vi "op_x2 Functional Test.vi"(0 "ENA1":bool caption="Connection 1 enable", 1 "IP address 1":string="172.16.14.23", 2 "ENA2":bool caption="Connection 2 enable", 3 "IP address 2":string="172.16.14.22", 4 "Operation text Refnum":refnum<vi>, 5 "error tick Refnum":refnum<vi>) -> ()   [LabVIEW 2015, in "VIPM2.lvlib"]
uses:
  VIPM2.lvlib
panel:
  out "Reports 2":string[](array[string])
  out "Reports 1":string[](array[string])
  in  "Close Button":bool
  in  "Execute Button":bool
  in  "Layers 2 cluster":T1(array[cluster]) {"LayerID" format="%x"}
  in  "All Layers 2":bool
  in  "Layers 1 cluster":T1(array[cluster]) {"LayerID" format="%x"}
  in  "All Layers 1":bool
  # "Select the Layers to execute the Functional Test"
  # "Bad pixels masked by software:\n      Chip D9EB: px 14\n      Chip 6B7B: px 60\n      Chip 3A65: px 00, 10, 20, 30, 40"
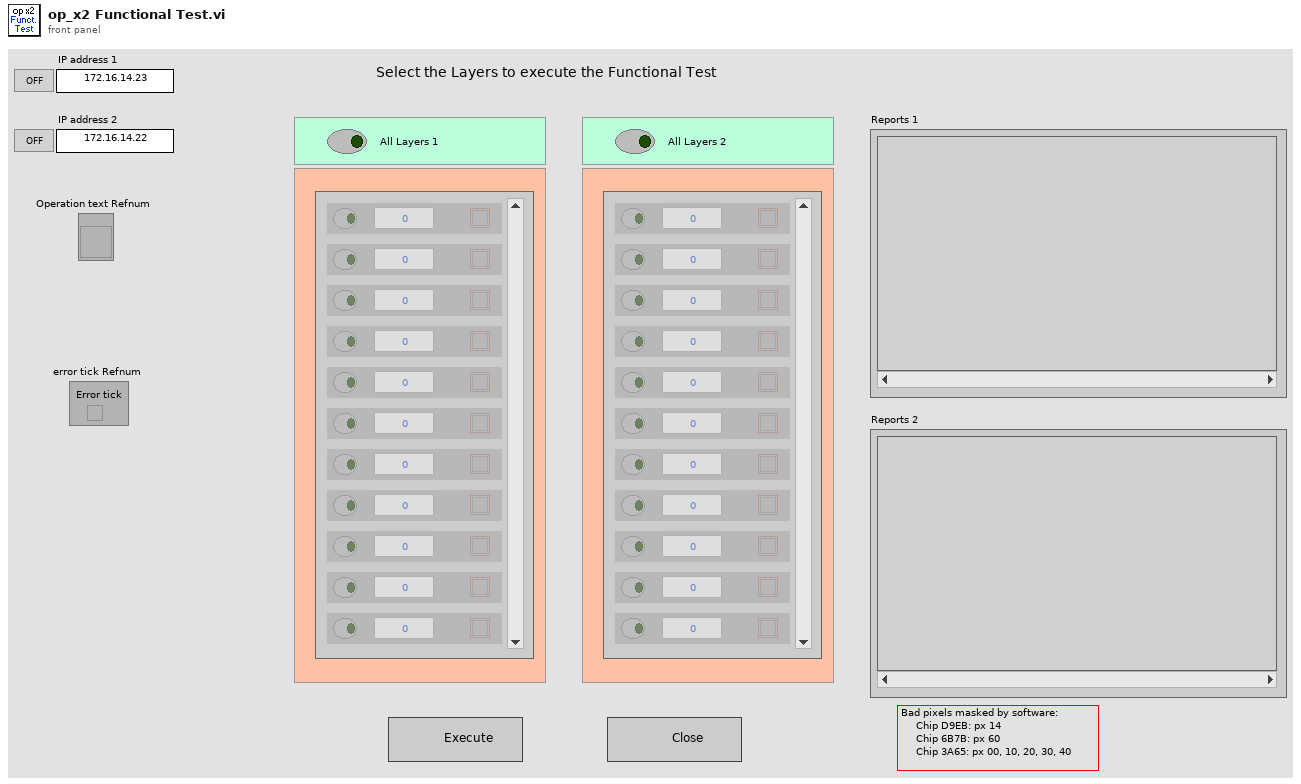
[diagram p1: front panel]
types:
  T1 = cluster{"Button":bool, "LayerID":u32, "Result":bool}[]
  T2 = cluster{"Button":bool, "LayerID":u32, "Result":bool}
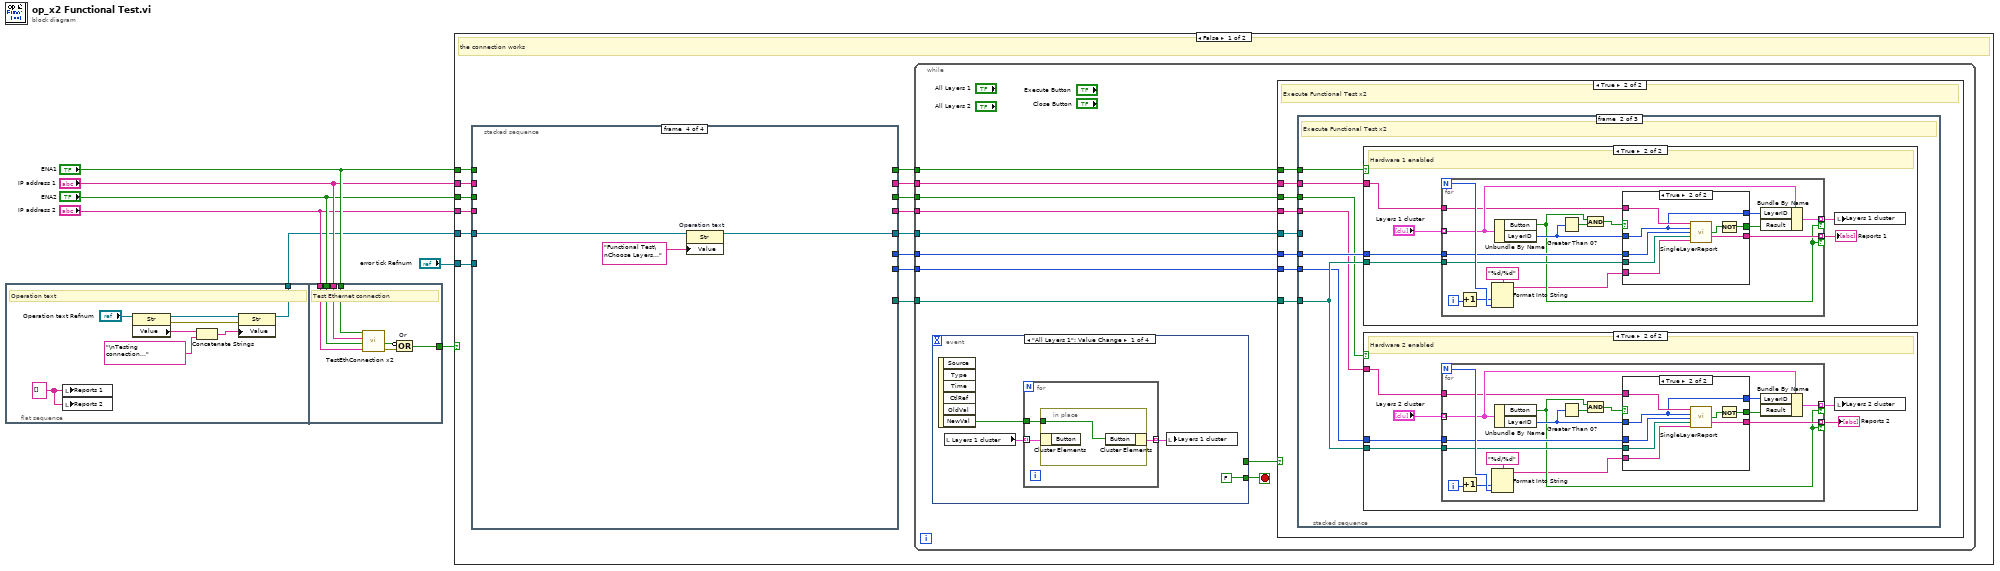
[diagram p0: block diagram]
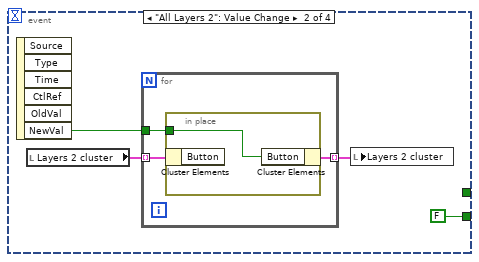
[diagram p2: hidden frame]
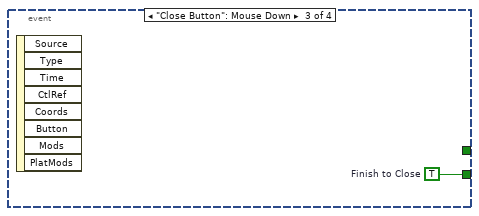
[diagram p3: hidden frame]
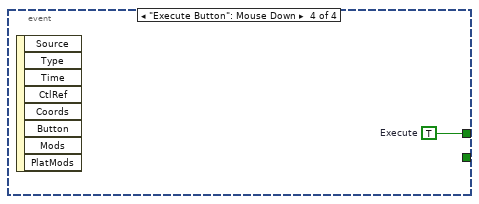
[diagram p4: hidden frame]
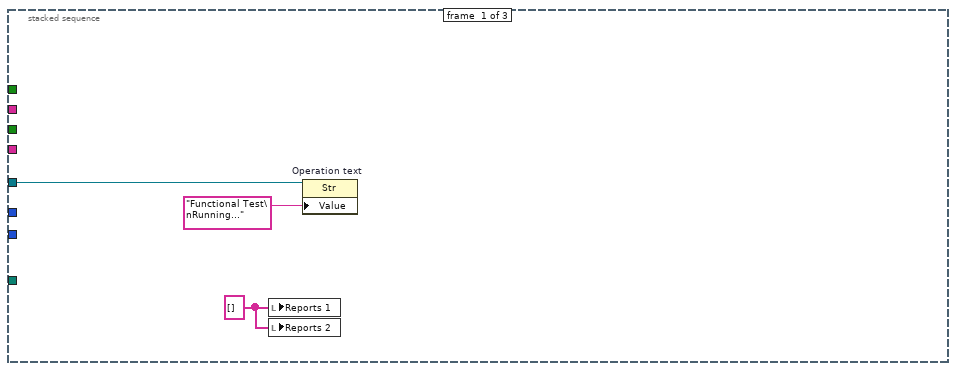
[diagram p6: hidden frame]
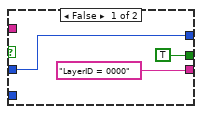
[diagram p8: hidden frame]
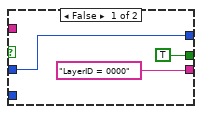
[diagram p10: hidden frame]
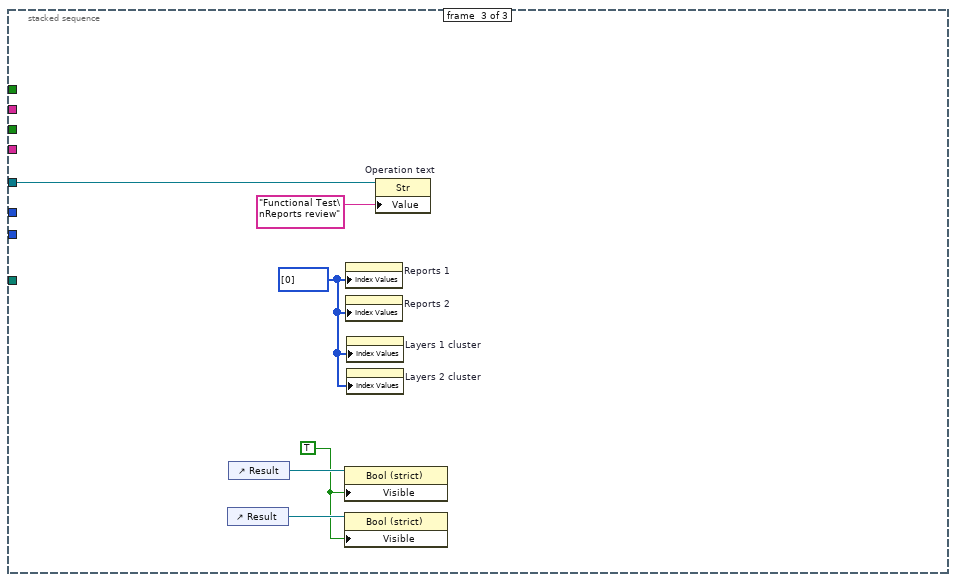
[diagram p11: hidden frame]
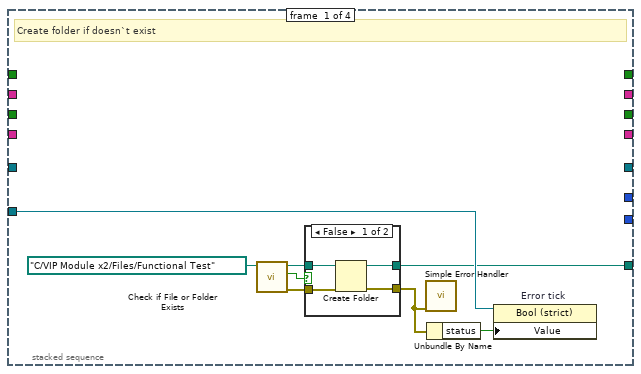
[diagram p12: hidden frame]
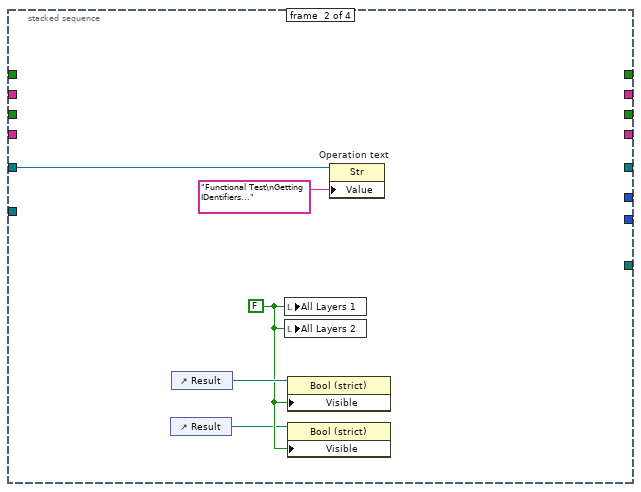
[diagram p14: hidden frame]
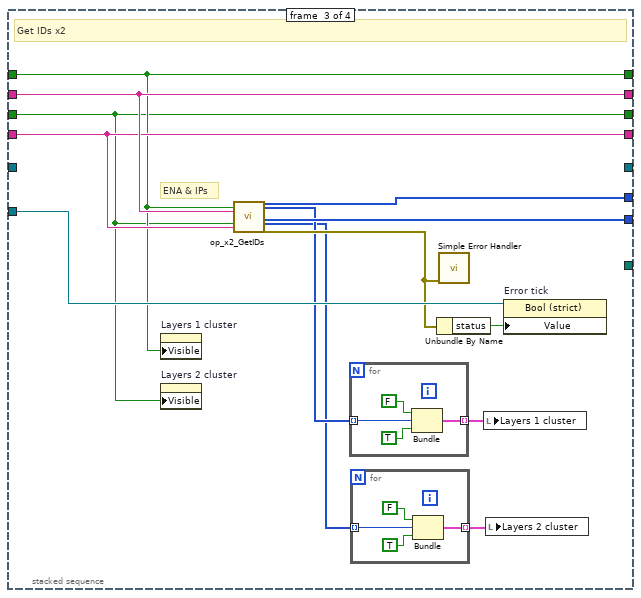
[diagram p15: hidden frame]
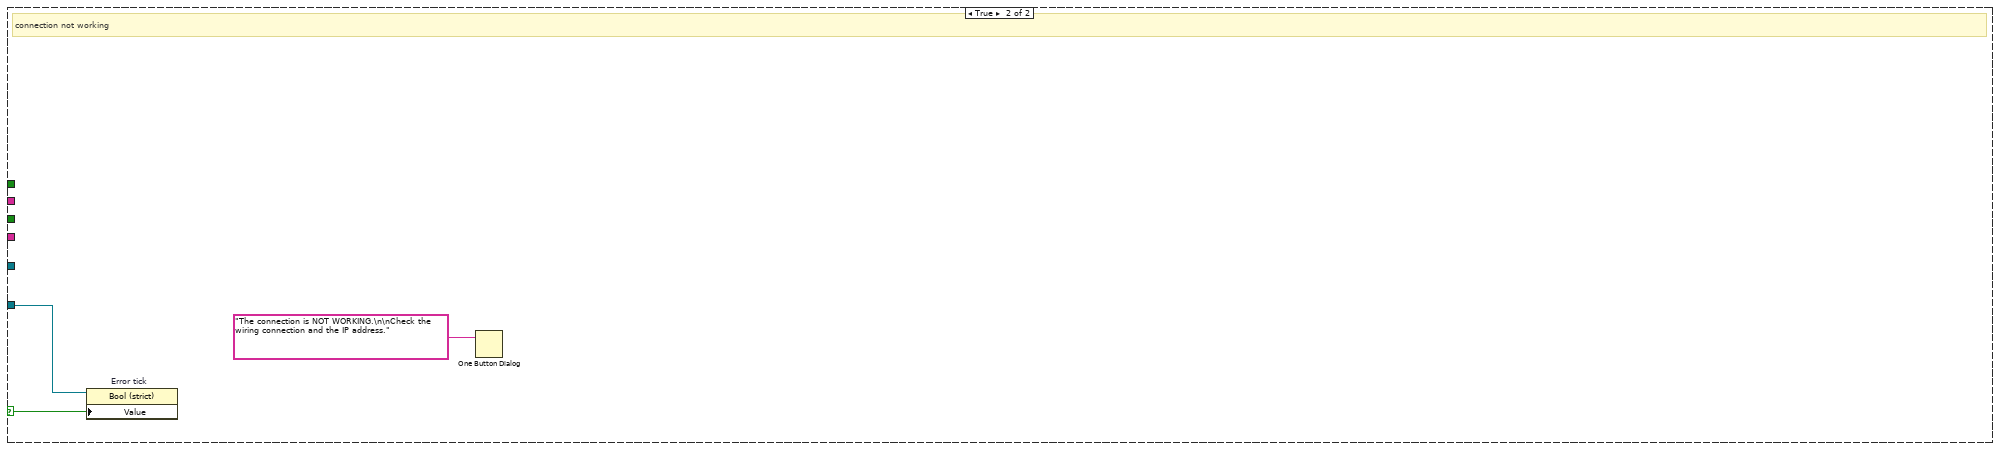
[diagram p16: hidden frame]
diagram:
  n1 = flat-sequence {
    tunnel: [w10] -> w1
    tunnel: "IP address 2" -> [w20]
    tunnel: "ENA2" -> [w19]
    tunnel: "IP address 1" -> [w18]
    tunnel: "ENA1" -> [w17]
    tunnel: [w16] -> w7
    frame #0 {
      w8 = string[] [] ("Reports 1")
      # "Operation text"
      n2 = local write "Reports 1"(w8) -> ()
      n3 = local write "Reports 2"(w8) -> ()
      n4 = property class="Str"(reference="Operation text Refnum") -> (reference out=w13:refnum<vi>, error out=w12:errorcluster, "Value"=w15:string)  [unwired: 1 in]
      n5 = Concatenate Strings "Concatenate Strings"(w15, "\nTesting connection..." ("string")) -> (w11:string)
      n6 = property class="Str"(reference=w13, error in=w12, "Value"=w11) -> (reference out=w10:refnum<vi>)  [unwired: 1 out]
    }
    frame #1 {
      # "Test Ethernet connection"
      n7 = call "TestEthConnection x2.vi"("IP address 2"=w20, "ENA2"=w19, "IP address 1"=w18, "ENA1"=w17) -> ("error out"=w21:errorcluster, "Answers OK?"=w22:bool)  [unwired: 6 in]
      n8 = Compound Arithmetic op=OR "Or"(invert w22, w21) -> (w16:bool)
    }
  }
  n9 = case shown="False" w7 {
    selector: w7 -> [_ w200]
    tunnel: "ENA1" -> [w35 _]
    tunnel: "IP address 1" -> [w34 _]
    tunnel: "error tick Refnum" -> [w36 w201]
    tunnel: "ENA2" -> [w33 _]
    tunnel: "IP address 2" -> [w32 _]
    tunnel: w1 -> [w31 _]
    frame False {
      # "the connection works"
      n10 = stacked-sequence {
        tunnel: w36 -> [w160 _ w188 _]
        tunnel: w35 -> [_ _ w177 _]
        tunnel: w34 -> [_ _ w179 _]
        tunnel: w33 -> [_ _ w176 _]
        tunnel: w32 -> [_ _ w178 _]
        tunnel: w31 -> [_ w175 _ w198]
        tunnel: [w157 _ _ _] -> w23
        tunnel: [_ _ w185 _] -> w25
        tunnel: [_ _ w184 _] -> w24
        tunnel: [_ _ _ w197] -> w26
        tunnel: [_ _ w177 _] -> w30
        tunnel: [_ _ w179 _] -> w29
        tunnel: [_ _ w176 _] -> w28
        tunnel: [_ _ w178 _] -> w27
        frame #0 {
          # "Create folder if doesn`t exist"
          n11 = call <vilib>:"Check if File or Folder Exists.vi"("path"=path "C:/VIP Module x2/Files/Functional Test") -> ("error out"=w162:errorcluster, "file or folder exists?"=w164:bool, "dup path"=w163:path)  [unwired: 8 in]
          n12 = case shown="False" w164 {
            tunnel: w163 -> [w168 w170]
            tunnel: [w167 w170] -> w157
            tunnel: w162 -> [w166 w169]
            tunnel: [w165 w169] -> w159
            frame False {
              n13 = Create Folder(path (use dialog)=w168, error in=w166) -> (created path=w167:path, error out=w165:errorcluster)  [unwired: 1 in, 1 out]
            }
            frame True {
            }
          }
          n14 = call <vilib>:"Simple Error Handler.vi"("error in (no error)"=w159) -> ()  [unwired: 4 in, 5 out]
          n15 = Unbundle By Name(w159) -> ("status"=w158:bool)
          n16 = property on="Error tick" class="Bool (strict)"(reference=w160, "Value"=w158) -> ()  [unwired: 1 in, 2 out]
        }
        frame #1 {
          w172 = FALSE ("All Layers 1")
          n17 = control-ref of="Result"() -> (w171:refnum<vi>)
          n18 = control-ref of="Result"() -> (w173:refnum<vi>)
          n19 = local write "All Layers 1"(w172) -> ()
          n20 = local write "All Layers 2"(w172) -> ()
          n21 = property class="Bool (strict)"(reference=w173, "Visible"=w172) -> ()  [unwired: 1 in, 2 out]
          n22 = property class="Bool (strict)"(reference=w171, "Visible"=w172) -> ()  [unwired: 1 in, 2 out]
          n23 = property on="Operation text" class="Str"(reference=w175, "Value"="Functional Test\nGetting IDentifiers...") -> ()  [unwired: 1 in, 2 out]
        }
        frame #2 {
          # "ENA & IPs"
          # "Get IDs x2"
          n24 = property on="Layers 1 cluster" class="Arr (strict)"("Visible"=w177) -> ()  [unwired: 2 in, 2 out]
          n25 = property on="Layers 2 cluster" class="Arr (strict)"("Visible"=w176) -> ()  [unwired: 2 in, 2 out]
          n26 = call "op_x2_GetIDs.vi"("ENA1"=w177, "IP address 1"=w179, "ENA2"=w176, "IP address 2"=w178) -> ("All ID list 1"=w185:u32[], "Layer ID list 1 (ordered)"=w182:u32[], "All ID list 2"=w184:u32[], "Layer ID list 2 (ordered)"=w181:u32[], "error out"=w186:errorcluster)  [unwired: 16 in, 3 out]
          n27 = for {
            tunnel: [w194] -> w183 mode=indexing
            tunnel: w182 -> [w193] mode=indexing
            n28 = Bundle(FALSE, w193, TRUE) -> (w194:cluster{bool, u32, bool})  [unwired: 1 in]
          }
          n29 = for {
            tunnel: [w190] -> w180 mode=indexing
            tunnel: w181 -> [w189] mode=indexing
            n30 = Bundle(FALSE, w189, TRUE) -> (w190:cluster{bool, u32, bool})  [unwired: 1 in]
          }
          n31 = Unbundle By Name(w186) -> ("status"=w187:bool)
          n32 = call <vilib>:"Simple Error Handler.vi"("error in (no error)"=w186) -> ()  [unwired: 4 in, 5 out]
          n33 = local write "Layers 1 cluster"(w183) -> ()
          n34 = local write "Layers 2 cluster"(w180) -> ()
          n35 = property on="Error tick" class="Bool (strict)"(reference=w188, "Value"=w187) -> ()  [unwired: 1 in, 2 out]
        }
        frame #3 {
          n36 = property on="Operation text" class="Str"(reference=w198, "Value"="Functional Test\nChoose Layers...") -> (reference out=w197:refnum<vi>)  [unwired: 1 in, 1 out]
        }
      }
      n37 = while {
        tunnel: w30 -> [w46]
        tunnel: w29 -> [w45]
        tunnel: w28 -> [w44]
        tunnel: w27 -> [w43]
        tunnel: w26 -> [w42]
        tunnel: w25 -> [w41]
        tunnel: w24 -> [w40]
        tunnel: w23 -> [w39]
        stop <- w37 stop-if-true
        n38 = event shown="[0] \"All Layers 1\": Value Change" {
          selector: _ -> [_ _ _ _]
          dyn-events: _ -> [_ _ _ _]
          timeout: _ -> [_ _ _ _]
          tunnel: [FALSE FALSE w63 _] -> w37
          tunnel: [_ _ _ w64] -> w38
          event "All Layers 1": Value Change {
            n39 = event-data() -> ("NewVal"=w49:bool)  [unwired: 1 in, 5 out]
            n40 = local read "Layers 1 cluster"() -> (w50:T1)
            n41 = for {
              tunnel: w50 -> [w53] mode=indexing
              tunnel: w49 -> [w52]
              tunnel: [w51] -> w48 mode=indexing
              n42 = in-place {
                in-place-border: w52 -> [w54]
                n43 = in-place-cluster #1(w53) -> ()  [unwired: 1 out]
                n44 = in-place-cluster #1("Button"=w54) -> (w51:T2)
              }
            }
            n45 = local write "Layers 1 cluster"(w48) -> ()
          }
          event "All Layers 2": Value Change {
            n46 = event-data() -> ("NewVal"=w57:bool)  [unwired: 1 in, 5 out]
            n47 = local read "Layers 2 cluster"() -> (w58:T1)
            n48 = for {
              tunnel: w58 -> [w61] mode=indexing
              tunnel: w57 -> [w60]
              tunnel: [w59] -> w56 mode=indexing
              n49 = in-place {
                in-place-border: w60 -> [w62]
                n50 = in-place-cluster #2(w61) -> ()  [unwired: 1 out]
                n51 = in-place-cluster #2("Button"=w62) -> (w59:T2)
              }
            }
            n52 = local write "Layers 2 cluster"(w56) -> ()
          }
          event "Close Button": Mouse Down {
            w63 = TRUE  # Finish to Close
            n53 = event-data() -> ()  [unwired: 1 in, 8 out]
          }
          event "Execute Button": Mouse Down {
            w64 = TRUE  # Execute
            n54 = event-data() -> ()  [unwired: 1 in, 8 out]
          }
        }
        n55 = case shown="True" w38 {
          tunnel: w46 -> [_ w71]
          tunnel: w45 -> [_ w70]
          tunnel: w44 -> [_ w69]
          tunnel: w43 -> [_ w68]
          tunnel: w42 -> [_ w72]
          tunnel: w41 -> [_ w67]
          tunnel: w40 -> [_ w65]
          tunnel: w39 -> [_ w66]
          frame False {
            # "No exe or Close"
          }
          frame True {
            # "Execute Functional Test x2"
            n56 = stacked-sequence {
              tunnel: w72 -> [w75 _ w155]
              tunnel: w71 -> [_ w82 _]
              tunnel: w70 -> [_ w81 _]
              tunnel: w69 -> [_ w76 _]
              tunnel: w68 -> [_ w77 _]
              tunnel: w67 -> [_ w80 _]
              tunnel: w66 -> [_ w79 _]
              tunnel: w65 -> [_ w78 _]
              frame #0 {
                w73 = string[] [] ("Reports 1")
                n57 = local write "Reports 1"(w73) -> ()
                n58 = local write "Reports 2"(w73) -> ()
                n59 = property on="Operation text" class="Str"(reference=w75, "Value"="Functional Test\nRunning...") -> ()  [unwired: 1 in, 2 out]
              }
              frame #1 {
                # "Execute Functional Test x2"
                n60 = case shown="True" w82 {
                  tunnel: w81 -> [_ w122]
                  tunnel: w80 -> [_ w121]
                  tunnel: w79 -> [_ w118]
                  frame False {
                    # "Hardware 1 not enabled"
                  }
                  frame True {
                    # "Hardware 1 enabled"
                    n61 = for {
                      N -> [w139]
                      tunnel: "Layers 1 cluster" -> [w138] mode=indexing
                      tunnel: w122 -> [w137]
                      tunnel: w121 -> [w136]
                      tunnel: [w133] -> w120 mode=indexing if=w128
                      tunnel: [w132] -> w119 mode=indexing if=w128
                      tunnel: w118 -> [w131]
                      i -> [w126]
                      n62 = Increment(x=w126) -> (x+1=w124:i32)
                      n63 = Format Into String(format string="%d/%d", w124, w139) -> (resulting string=w123:string)  [unwired: 2 in, 1 out]
                      n64 = Unbundle By Name(w138) -> ("Button"=w128:bool, "LayerID"=w130:u32)
                      n65 = Greater Than 0?(x=w130) -> (x > 0?=w129:bool)
                      n66 = And(x=w128, y=w129) -> (x .and. y?=w127:bool)
                      n67 = case shown="True" w127 {
                        tunnel: w137 -> [_ w150]
                        tunnel: w130 -> [w142 w146]
                        tunnel: w136 -> [_ w145]
                        tunnel: [w142 w146] -> w135
                        tunnel: [TRUE w148] -> w134
                        tunnel: ["LayerID = 0000" ("Report out") w147] -> w132
                        tunnel: w131 -> [_ w144]
                        tunnel: w123 -> [_ w143]
                        frame False {
                        }
                        frame True {
                          n68 = call "SingleLayerReport.vi"("IP address"=w150, "LayerID under test"=w146, "All ID list"=w145, "Report folder path"=w144, "process"=w143) -> ("Test OK?"=w149:bool, "Report out"=w147:string)  [unwired: 7 in, 2 out]
                          n69 = Not(x=w149) -> (.not. x?=w148:bool)
                        }
                      }
                      n70 = Bundle By Name(cluster=w138, "LayerID"=w135, "Result"=w134) -> (w133:T2)
                    }
                    "Reports 1" <- w119
                    n71 = local write "Layers 1 cluster"(w120) -> ()
                  }
                }
                n72 = case shown="True" w76 {
                  tunnel: w77 -> [_ w88]
                  tunnel: w78 -> [_ w87]
                  tunnel: w79 -> [_ w85]
                  frame False {
                    # "Hardware 2 not enabled"
                  }
                  frame True {
                    # "Hardware 2 enabled"
                    n73 = for {
                      N -> [w105]
                      tunnel: "Layers 2 cluster" -> [w104] mode=indexing
                      tunnel: w88 -> [w103]
                      tunnel: w87 -> [w102]
                      tunnel: [w99] -> w86 mode=indexing if=w94
                      tunnel: [w98] -> w84 mode=indexing if=w94
                      tunnel: w85 -> [w97]
                      i -> [w92]
                      n74 = Increment(x=w92) -> (x+1=w90:i32)
                      n75 = Format Into String(format string="%d/%d", w90, w105) -> (resulting string=w89:string)  [unwired: 2 in, 1 out]
                      n76 = Unbundle By Name(w104) -> ("Button"=w94:bool, "LayerID"=w96:u32)
                      n77 = Greater Than 0?(x=w96) -> (x > 0?=w95:bool)
                      n78 = And(x=w94, y=w95) -> (x .and. y?=w93:bool)
                      n79 = case shown="True" w93 {
                        tunnel: w103 -> [_ w116]
                        tunnel: w96 -> [w108 w112]
                        tunnel: w102 -> [_ w111]
                        tunnel: [w108 w112] -> w101
                        tunnel: [TRUE w114] -> w100
                        tunnel: ["LayerID = 0000" ("Report out") w113] -> w98
                        tunnel: w97 -> [_ w110]
                        tunnel: w89 -> [_ w109]
                        frame False {
                        }
                        frame True {
                          n80 = call "SingleLayerReport.vi"("IP address"=w116, "LayerID under test"=w112, "All ID list"=w111, "Report folder path"=w110, "process"=w109) -> ("Test OK?"=w115:bool, "Report out"=w113:string)  [unwired: 7 in, 2 out]
                          n81 = Not(x=w115) -> (.not. x?=w114:bool)
                        }
                      }
                      n82 = Bundle By Name(cluster=w104, "LayerID"=w101, "Result"=w100) -> (w99:T2)
                    }
                    "Reports 2" <- w84
                    n83 = local write "Layers 2 cluster"(w86) -> ()
                  }
                }
              }
              frame #2 {
                w151 = u32[] [0] ("Index Values")
                w152 = TRUE
                n84 = control-ref of="Result"() -> (w154:refnum<vi>)
                n85 = control-ref of="Result"() -> (w153:refnum<vi>)
                n86 = property class="Bool (strict)"(reference=w153, "Visible"=w152) -> ()  [unwired: 1 in, 2 out]
                n87 = property class="Bool (strict)"(reference=w154, "Visible"=w152) -> ()  [unwired: 1 in, 2 out]
                n88 = property on="Reports 1" class="Arr (strict)"("Index Values"=w151) -> ()  [unwired: 2 in, 2 out]
                n89 = property on="Reports 2" class="Arr (strict)"("Index Values"=w151) -> ()  [unwired: 2 in, 2 out]
                n90 = property on="Layers 1 cluster" class="Arr (strict)"("Index Values"=w151) -> ()  [unwired: 2 in, 2 out]
                n91 = property on="Layers 2 cluster" class="Arr (strict)"("Index Values"=w151) -> ()  [unwired: 2 in, 2 out]
                n92 = property on="Operation text" class="Str"(reference=w155, "Value"="Functional Test\nReports review") -> ()  [unwired: 1 in, 2 out]
              }
            }
          }
        }
      }
    }
    frame True {
      # "connection not working"
      n93 = property on="Error tick" class="Bool (strict)"(reference=w201, "Value"=w200) -> ()  [unwired: 1 in, 2 out]
      n94 = One Button Dialog(message="The connection is NOT WORKING.\n\nCheck the wiring connection and the IP address.") -> ()  [unwired: 1 in, 1 out]
    }
  }
